vi "Read Measurement (Current Value).vi"(0 "VISA resource name":refnum<visa-resource-name>, 1 "Slope Type (0: Positive)":i32(ring) items=["Positive", "Negative"], 5 "Measurement Type (0: Peak-Peak)":i32(ring) items=["Peak-Peak", "Maximum", "Minimum", "Amplitude", "Top", "Base", "Overshoot", "Preshoot", "Average - N Cycles", "Average - Full Screen", "DC RMS - N Cycles", "DC RMS - Full Screen", "AC RMS - N Cycles", "AC RMS - Full Screen (Std Dev)", "Ratio", "Period", "Frequency", "Counter", "+Width", "-Width", "Burst Width", "Duty Cycle", "Rise Time", "Fall Time", "Delay", "Phase", "X minY", "X maxY", "Positive Pulse Count", "Negative Pulse Count", "Raising Edge Count", "Falling Edge Count", "Area - N Cycle", "Area - Full Screen", "Nth Edge Time", "Nth Edge Cross Level Time"], 7 "Occurrence Value (1)":i32=1, 9 "Vertical Cross Value (0)":dbl, 11 "error in (no error)":errorcluster) -> (4 "VISA resource name out":refnum<visa-resource-name>, 6 "Result Value":dbl, 15 "error out":errorcluster)   [LabVIEW 2023, in "Keysight-DSQx3014T.lvlib"]
doc: "Returns the measurement of continoues acquisition."
uses:
  Keysight-DSQx3014T.lvlib
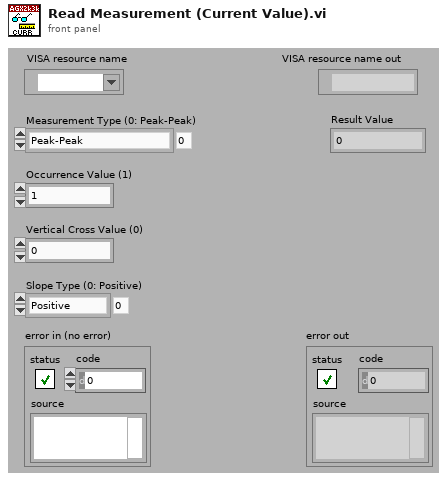
[diagram p1: front panel]
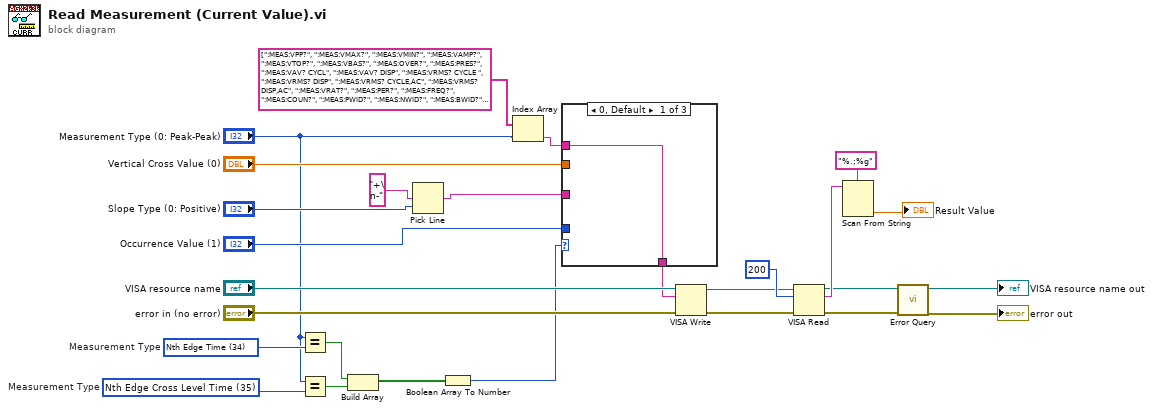
[diagram p0: block diagram]
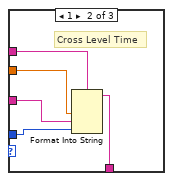
[diagram p2: hidden frame]
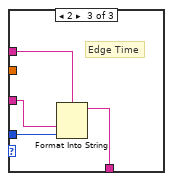
[diagram p3: hidden frame]
diagram:
  w15 = 35 items=["Peak-Peak", "Maximum", "Mimimum", "Amplitude", "Top", "Base", "Overshoot", "Preshoot", "Average - N Cycles", "Average - Full Screen", "DC RMS - N Cycles", "DC RMS - Full Screen", "AC RMS - N Cycles", "AC RMS - Full Screen (Std Dev)", "Ratio", "Period", "Frequency", "Counter", "+Width", "-Width", "Burst Width", "Duty Cycle", "Rise Time", "Fall Time", "Delay", "Phase", "X minY", "X maxY", "Positive Pulse Count", "Negative Pulse Count", "Raising Edge Count", "Falling Edge Count", "Area - N Cycle", "Area - Full Screen", "Nth Edge Time", "Nth Edge Cross Level Time"]  # Measurement Type
  w14 = 34 items=["Peak-Peak", "Maximum", "Mimimum", "Amplitude", "Top", "Base", "Overshoot", "Preshoot", "Average - N Cycles", "Average - Full Screen", "DC RMS - N Cycles", "DC RMS - Full Screen", "AC RMS - N Cycles", "AC RMS - Full Screen (Std Dev)", "Ratio", "Period", "Frequency", "Counter", "+Width", "-Width", "Burst Width", "Duty Cycle", "Rise Time", "Fall Time", "Delay", "Phase", "X minY", "X maxY", "Positive Pulse Count", "Negative Pulse Count", "Raising Edge Count", "Falling Edge Count", "Area - N Cycle", "Area - Full Screen", "Nth Edge Time", "Nth Edge Cross Level Time"]  # Measurement Type
  n1 = Equal?(x="Measurement Type (0: Peak-Peak)", y=w14) -> (x = y?=w12:bool)
  n2 = Equal?(x="Measurement Type (0: Peak-Peak)", y=w15) -> (x = y?=w11:bool)
  n3 = Build Array(w12, w11) -> (w10:bool[])
  n4 = Pick Line(multi-line string="+\n-", line index="Slope Type (0: Positive)") -> (output string=w4:string)  [unwired: 1 out]
  n5 = Boolean Array To Number(Boolean array=w10) -> (number=w9:u32)
  n6 = Index Array(array=string[] [":MEAS:VPP?", ":MEAS:VMAX?", ":MEAS:VMIN?", ":MEAS:VAMP?", ":MEAS:VTOP?", ":MEAS:VBAS?", ":MEAS:OVER?", ":MEAS:PRES?", ":MEAS:VAV? CYCL", ":MEAS:VAV? DISP", ":MEAS:VRMS? CYCLE ", ":MEAS:VRMS? DISP", ":MEAS:VRMS? CYCLE,AC", ":MEAS:VRMS? DISP,AC", ":MEAS:VRAT?", ":MEAS:PER?", ":MEAS:FREQ?", ":MEAS:COUN?", ":MEAS:PWID?", ":MEAS:NWID?", ":MEAS:BWID?", ":MEAS:DUTY?", ":MEAS:RIS?", ":MEAS:FALL?", ":MEAS:DEL?", ":MEAS:PHAS?", ":MEAS:XMIN?", ":MEAS:XMAX?", ":MEAS:PPUL?", ":MEAS:NPUL?", ":MEAS:PEDG?", ":MEAS:NEDG?", ":MEAS:ARE?", ":MEAS:ARE?", "%.;:MEAS:TEDG? %s%d", "%.;:MEAS:TVAL? %g, %s%d"] ("Array"), index="Measurement Type (0: Peak-Peak)") -> (element=w3:string)
  n7 = case shown="0, Default" w9 {
    tunnel: w3 -> [w28 w30 w37]
    tunnel: [w28 w29 w34] -> w13
    tunnel: "Vertical Cross Value (0)" -> [_ w33 _]
    tunnel: w4 -> [_ w32 w36]
    tunnel: "Occurrence Value (1)" -> [_ w31 w35]
    frame 0, Default {
    }
    frame 1 {
      # "Cross Level Time"
      n8 = Format Into String(format string=w30, w33, w32, w31) -> (resulting string=w29:string)  [unwired: 2 in, 1 out]
    }
    frame 2 {
      # "Edge Time"
      n9 = Format Into String(format string=w37, w36, w35) -> (resulting string=w34:string)  [unwired: 2 in, 1 out]
    }
  }
  n10 = VISA Write(VISA resource name="VISA resource name", write buffer=w13, error in (no error)="error in (no error)") -> (VISA resource name out=w20:refnum<visa-resource-name>, error out=w19:errorcluster)  [unwired: 1 out]
  n11 = VISA Read(VISA resource name=w20, byte count=u32 200, error in (no error)=w19) -> (VISA resource name out=w18:refnum<visa-resource-name>, read buffer=w22:string, error out=w17:errorcluster)  [unwired: 1 out]
  n12 = Scan From String(format string="%.;%g", input string=w22) -> (output 1=→"Result Value":dbl)  [unwired: 2 in, 4 out]
  n13 = call "Error Query.vi"("error in (no error)"=w17, "VISA resource name"=w18) -> ("error out"=→"error out":errorcluster, "VISA resource name out"=→"VISA resource name out":refnum<visa-resource-name>)  [unwired: 8 out]
